vi "evo_irimager_set_focusmotor_pos.vi"(11 "Focus Pos %":sgl min=0 max=100) -> (3 "function return":i32)   [LabVIEW 2017, in "libirimager_direct_binding.lvlib"]
uses:
  libirimager_direct_binding.lvlib
  labview/libirimager.dll
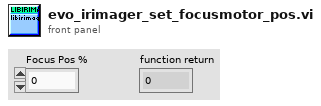
[diagram p1: front panel]
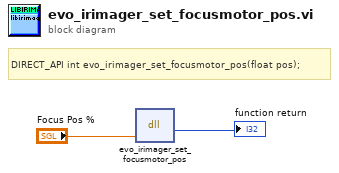
[diagram p0: block diagram]
diagram:
  # "DIRECT_API int evo_irimager_set_focusmotor_pos(float pos);"
  n1 = dll-call lib="C:/Users/HelmutEngelhardt/Documents/labview/libirimager.dll" fn="evo_irimager_set_focusmotor_pos"("pos"="Focus Pos %") -> ("Rückgabetyp"=→"function return":i32)  [unwired: 4 in, 2 out]
